vi "UTC Unix Time.vi"() -> (1 "Fractional Second":dbl, 2 "Unix Time (s)":u64)   [LabVIEW 2010]
panel:
  # "Returns current time in \nUnix UTC format 64-bit\nwhole second and fractional\nsecond."
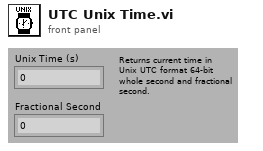
[diagram p1: front panel]
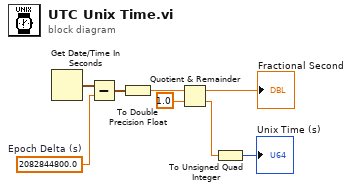
[diagram p0: block diagram]
diagram:
  w7 = 2082844800.0  # Epoch Delta (s)
  n1 = Get Date/Time In Seconds() -> (seconds since 1Jan1904=w8:timestamp)
  n2 = Subtract(x=w8, y=w7) -> (x-y=w6:timestamp)
  n3 = To Double Precision Float(number=w6) -> (double precision float=w5:dbl)
  n4 = Quotient & Remainder(x=w5, y=1.0) -> (x-y*floor(x/y)=→"Fractional Second":dbl, floor(x/y)=w2:dbl)
  n5 = To Unsigned Quad Integer(1:w2) -> (0:→"Unix Time (s)":u64)
